vi "MES_Local_SoftFP.vi"(0 "reference in":refnum<class "MES_Local.lvclass">, 2 "Floating":bool, 5 "error in (no error)":errorcluster) -> (14 "reference out":refnum<class "MES_Local.lvclass">, 19 "error out":errorcluster)   [LabVIEW 2022 SP3, in "MES_Local.lvlib" / "MES_Local.lvclass"]
uses:
  MES_Local.lvclass
  Components/ViPER.lvlibp/ViPER.lvclass
  C:/Projects/Medulla/ViPER/Examples/Flux_Capacitor_Tester/Components/ViPER.lvlibp/ViPER.lvclass
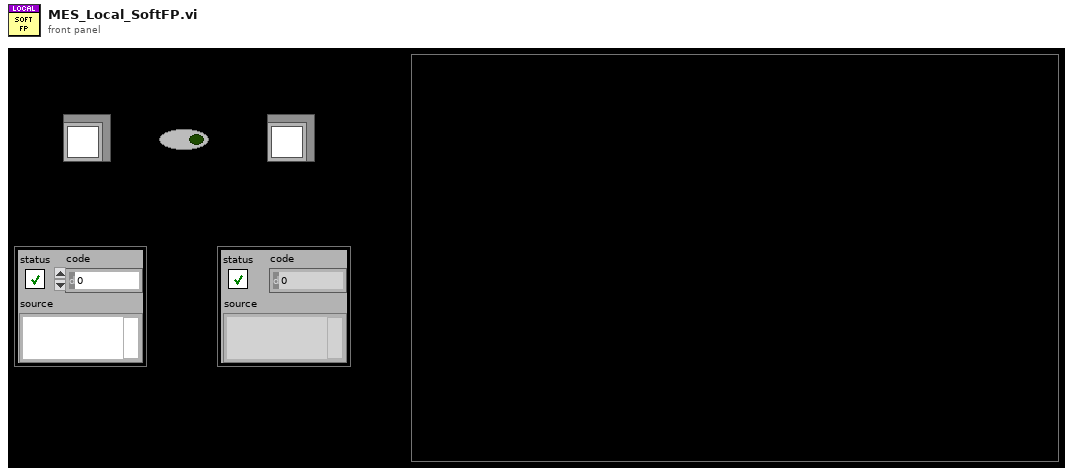
[diagram p1: front panel]
types:
  T1 = enum32{"Invalid", "Standard", "Closed", "Hidden", "Minimized", "Maximized"}
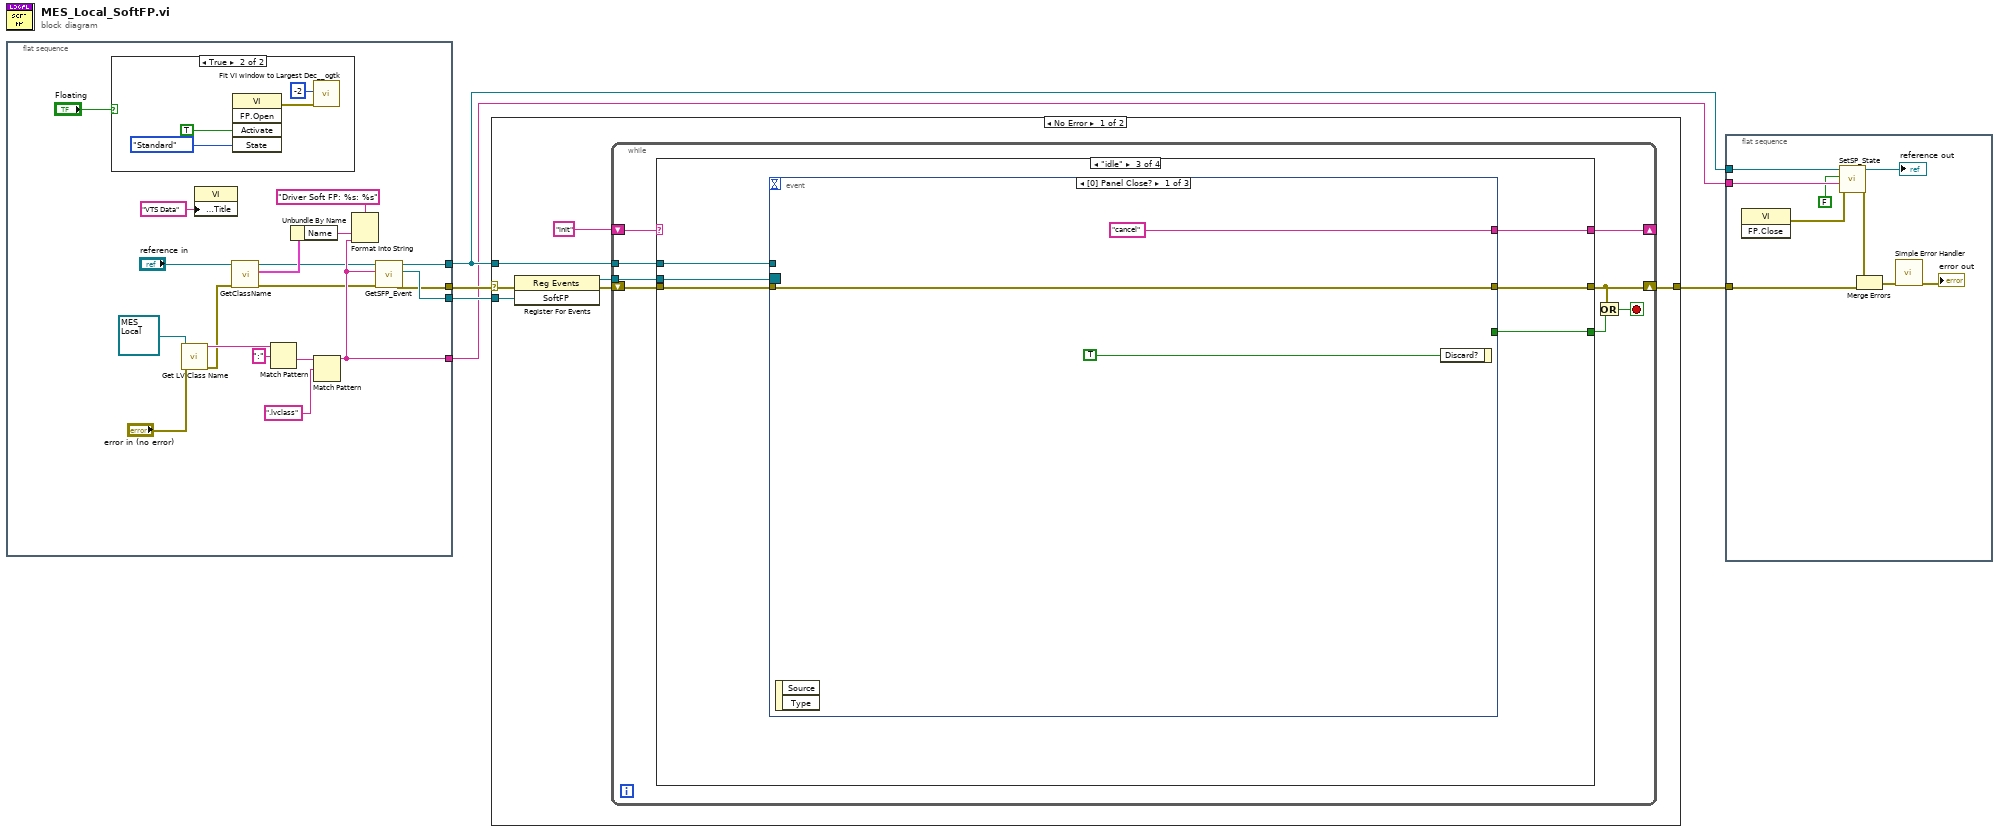
[diagram p0: block diagram]
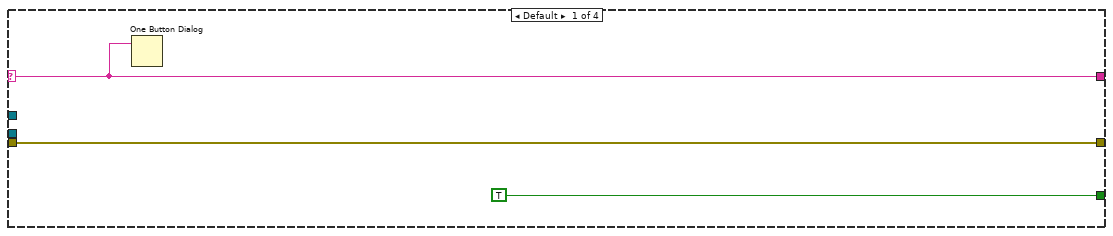
[diagram p3: hidden frame]
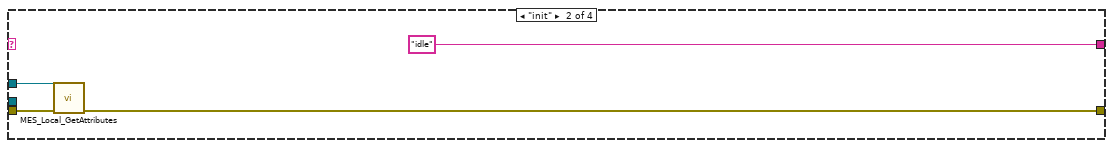
[diagram p4: hidden frame]
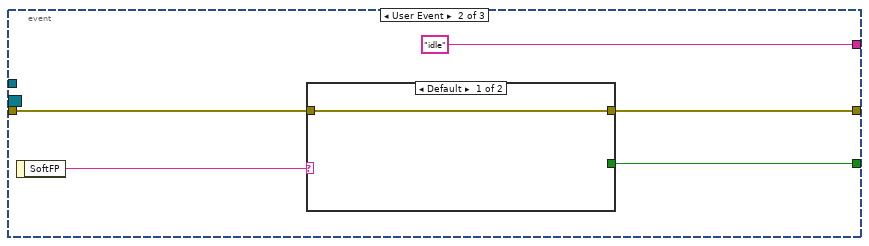
[diagram p5: hidden frame]
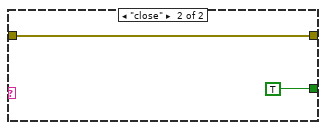
[diagram p6: hidden frame]
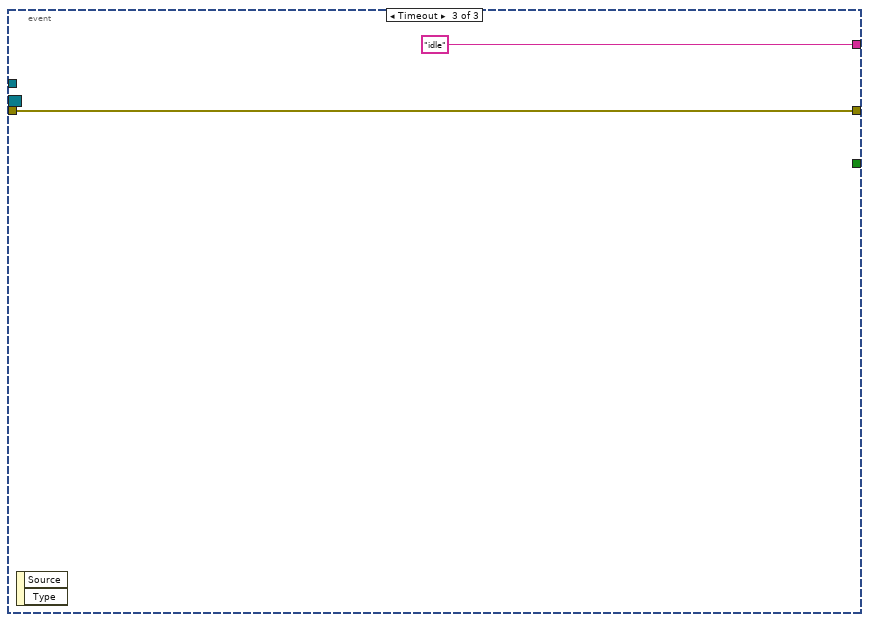
[diagram p7: hidden frame]
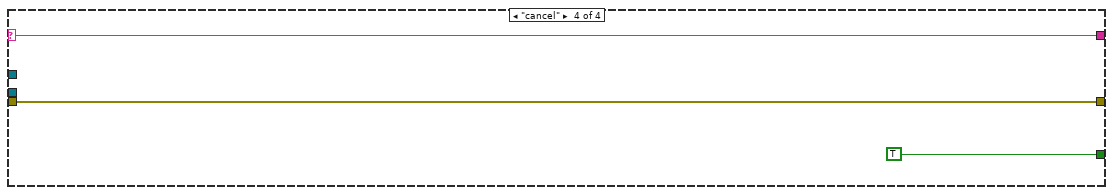
[diagram p8: hidden frame]
diagram:
  n1 = flat-sequence {
    tunnel: [w22] -> w5
    tunnel: [w21] -> w2
    tunnel: [w24] -> w3
    tunnel: [w13] -> w1
    frame #0 {
      n2 = case shown="True" "Floating" {
        frame False {
        }
        frame True {
          n3 = invoke class="VI" method="FP.Open"("Activate"=TRUE ("Activate?"), "State"=T1."Standard") -> (error out=w25:errorcluster)  [unwired: 3 in, 4 out]
          n4 = call <userlib>:"Fit VI window to Largest Dec__ogtk.vi"("error in (no error)"=w25, "border spacing (2 px)"=-2) -> ()  [unwired: 4 in, 2 out]
        }
      }
      n5 = call <vilib>:"Get LV Class Name.vi"("error in (no error)"="error in (no error)", "object"=refnum<class "MES_Local.lvclass"> refnum ("reference")) -> ("error out"=w12:errorcluster, "class name"=w18:string)  [unwired: 8 in]
      n6 = property class="VI"("Front Panel.Title"="VTS Data" ("Front Panel Window:Title")) -> ()  [unwired: 2 in, 2 out]
      n7 = call "GetClassName.vi"("error in (no error)"=w12, "reference in"="reference in") -> ("error out"=w11:errorcluster, "Details"=w10:cluster{"Name":string, "Class":string}, "reference out"=w8:refnum<class "MES_Local.lvclass">)  [unwired: 7 in]
      n8 = Match Pattern(string=w18, regular expression=":") -> (after substring=w16:string)  [unwired: 1 in, 3 out]
      n9 = Unbundle By Name(w10) -> ("Name"=w20:string)
      n10 = Match Pattern(string=w16, regular expression=".lvclass") -> (before substring=w13:string)  [unwired: 1 in, 3 out]
      n11 = Format Into String(format string="Driver Soft FP: %s: %s", w20, w13) -> ()  [unwired: 2 in, 2 out]
      n12 = call-dynamic "GetSFP_Event.vi"("error in (no error)"=w11, "Ancestor"=w13, "reference in"=w8) -> ("error out"=w22:errorcluster, "SoftFP"=w24:refnum<user-event>, "reference out"=w21:refnum<class "MES_Local.lvclass">)  [unwired: 6 in]
    }
  }
  n13 = case shown="No Error" w5 {
    selector: w5 -> [w33 w73]
    tunnel: [w29 w73] -> w4
    tunnel: w2 -> [w30 _]
    tunnel: w3 -> [w35 _]
    frame No Error {
      n14 = register-events(error in=w33, w35) -> (reference out=w34:refnum<event-registration>, error out=w32:errorcluster)  [unwired: 1 in]
      n15 = while {
        shift-right: [w40] -> w29
        shift-left: w32 -> [w43]
        tunnel: w34 -> [w42]
        tunnel: w30 -> [w41]
        shift-right: [w36] -> _
        shift-left: "init" -> [w37]
        stop <- w39 stop-if-true
        n16 = case shown="\"idle\"" w37 {
          selector: w37 -> [w44 _ _ w71]
          tunnel: w43 -> [w45 w49 w56 w70]
          tunnel: w42 -> [_ _ w55 _]
          tunnel: w41 -> [_ w48 w54 _]
          tunnel: [w45 w47 w53 w70] -> w40
          tunnel: [TRUE ("Discard?") _ w52 TRUE ("OK")] -> w38
          tunnel: [w44 "idle" w51 w71] -> w36
          frame Default {
            n17 = One Button Dialog(message=w44) -> ()  [unwired: 1 in, 1 out]
          }
          frame "init" {
            n18 = call "MES_Local_GetAttributes.vi"("error in (no error)"=w49, "reference in"=w48) -> ("error out"=w47:errorcluster)  [unwired: 6 in, 3 out]
          }
          frame "idle" {
            n19 = event shown="[0] Panel Close?" {
              selector: w55 -> [_ _ _]
              dyn-events: _ -> [_ _ _]
              timeout: _ -> [_ _ _]
              tunnel: w56 -> [w59 w64 w69]
              tunnel: [w59 w62 w69] -> w53
              tunnel: [_ w61 _] -> w52
              tunnel: w54 -> [_ _ _]
              tunnel: ["cancel" "idle" "idle"] -> w51
              event Panel Close? {
                n20 = event-data() -> ()  [unwired: 1 in, 2 out]
                n21 = event-data("Discard?"=TRUE) -> ()  [unwired: 1 in, 1 out]
              }
              event User Event {
                n22 = event-data() -> ("SoftFP"=w63:string)  [unwired: 1 in]
                n23 = case shown="Default" w63 {
                  tunnel: w64 -> [w65 w67]
                  tunnel: [w65 w67] -> w62
                  tunnel: [_ TRUE ("Discard?")] -> w61
                  frame Default {
                  }
                  frame "close" {
                  }
                }
              }
              event Timeout {
                n24 = event-data() -> ()  [unwired: 1 in, 2 out]
              }
            }
          }
          frame "cancel" {
          }
        }
        n25 = Or(x=w40, y=w38) -> (x .or. y?=w39:bool)
      }
    }
    frame Error {
    }
  }
  n26 = flat-sequence {
    tunnel: w4 -> [w80]
    tunnel: w2 -> [w75]
    tunnel: w1 -> [w77]
    frame #0 {
      n27 = invoke class="VI" method="FP.Close"() -> (error out=w79:errorcluster)  [unwired: 3 in, 2 out]
      n28 = call "SetSP_State.vi"("error in (no error)"=w79, "Ancestor"=w77, "SP Open"=FALSE, "reference in"=w75) -> ("error out"=w78:errorcluster, "reference out"=→"reference out":refnum<class "MES_Local.lvclass">)  [unwired: 6 in]
      n29 = Merge Errors(w78, w80) -> (w82:errorcluster)
      n30 = call <vilib>:"Simple Error Handler.vi"("error in (no error)"=w82) -> ("error out"=→"error out":errorcluster)  [unwired: 4 in, 4 out]
    }
  }
